vi "NI-DAQmx.vi"() -> (15 "error out":errorcluster)   [LabVIEW 2013]
uses:
  <vilib>/DAQmx/read.llb/DAQmx Read (Analog 2D DBL NChan NSamp).vi
  Globals/Meas_global.vi
  PWA/PWAtasksGLOBAL.vi
  <vilib>/DAQmx/configure/timing.llb/DAQmx Timing (Sample Clock).vi
  <vilib>/DAQmx/miscellaneous.llb/DAQmx Fill In Error Info.vi
  <resource>/objmgr/daqmx.rc
panel:
  out "CurrReadPos 2":dbl=1024.0
  out "AvailSampPerChan 2":u32
  out "TotalSampPerChanAcquired 2":dbl=1024.0
  out "AuditTrail":string[](array[string])
  out "TotalSampPerChanAcquired":dbl=1024.0
  out "AvailSampPerChan":u32
  out "CurrReadPos":dbl=1024.0
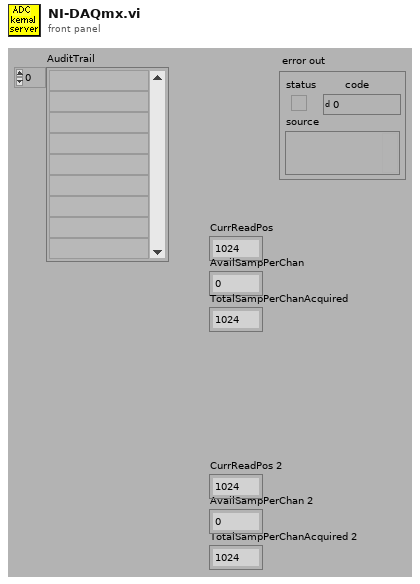
[diagram p1: front panel]
types:
  T1 = typedef "Ch_and_Spans.ctl" = cluster{"high limit (10V)":sgl, "low limit (-10V)":sgl, "Ch No":i16, "Var name":string, "Use Latest Calib":bool, "DAQmx Chan":tag}
  T2 = typedef "LDA_Setup.ctl" = cluster{"dimensions":enum16{"1D", "2D"}, "Analogue Freq Multiplier":dbl}
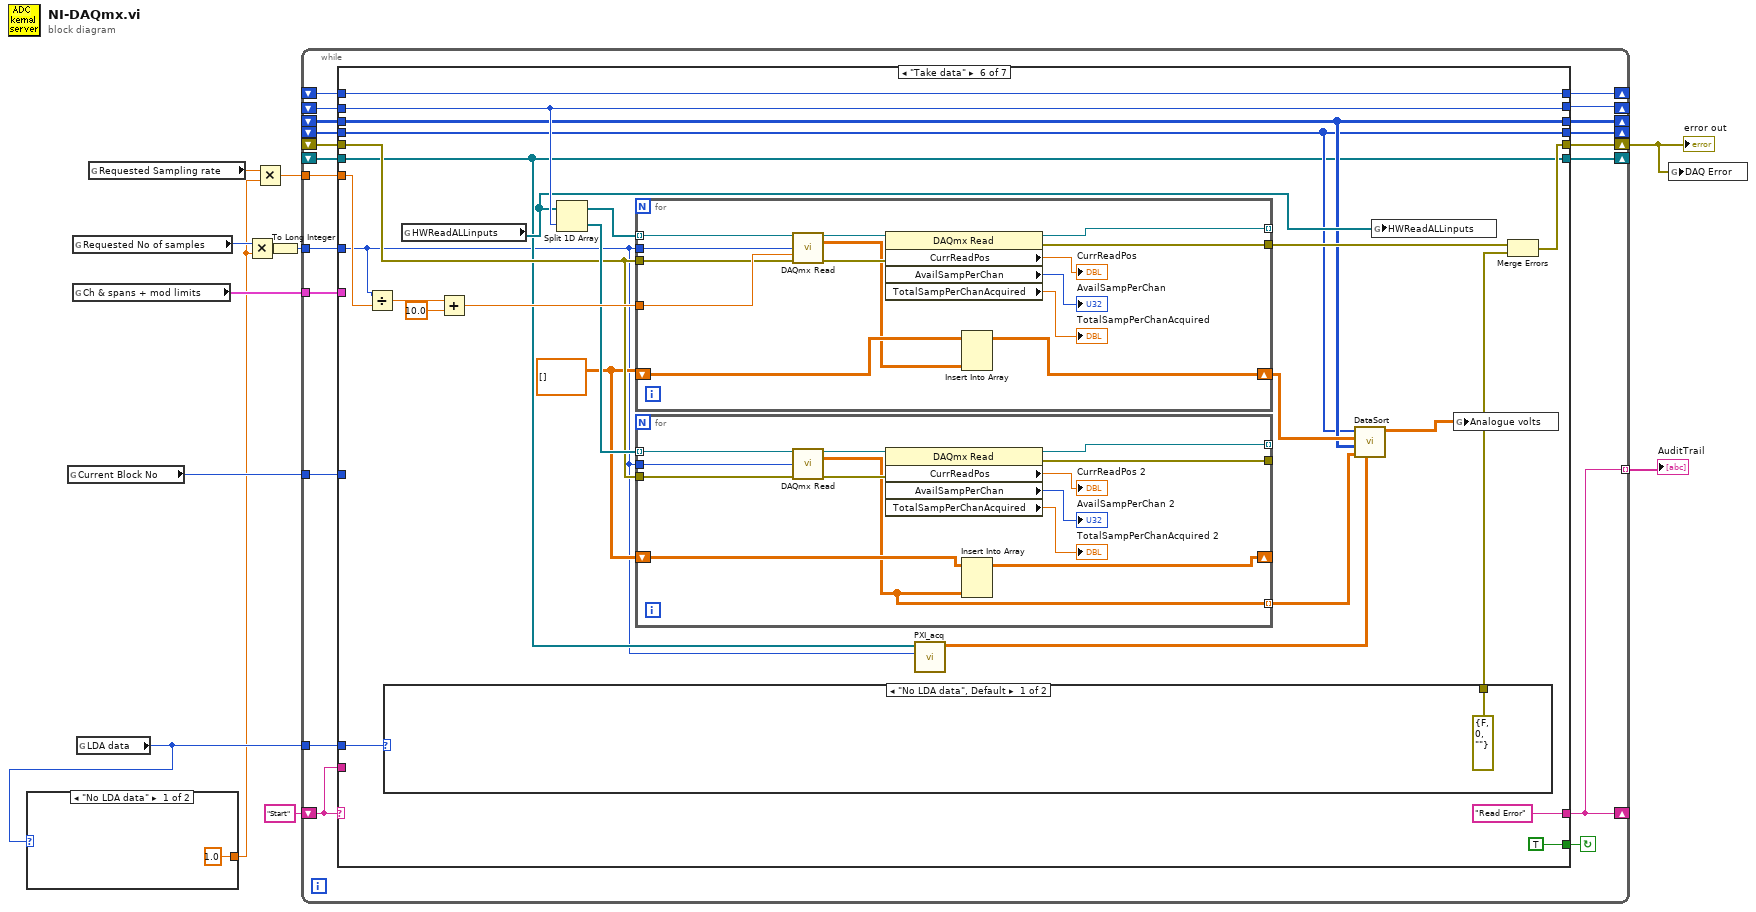
[diagram p0: block diagram]
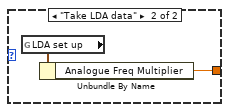
[diagram p2: hidden frame]
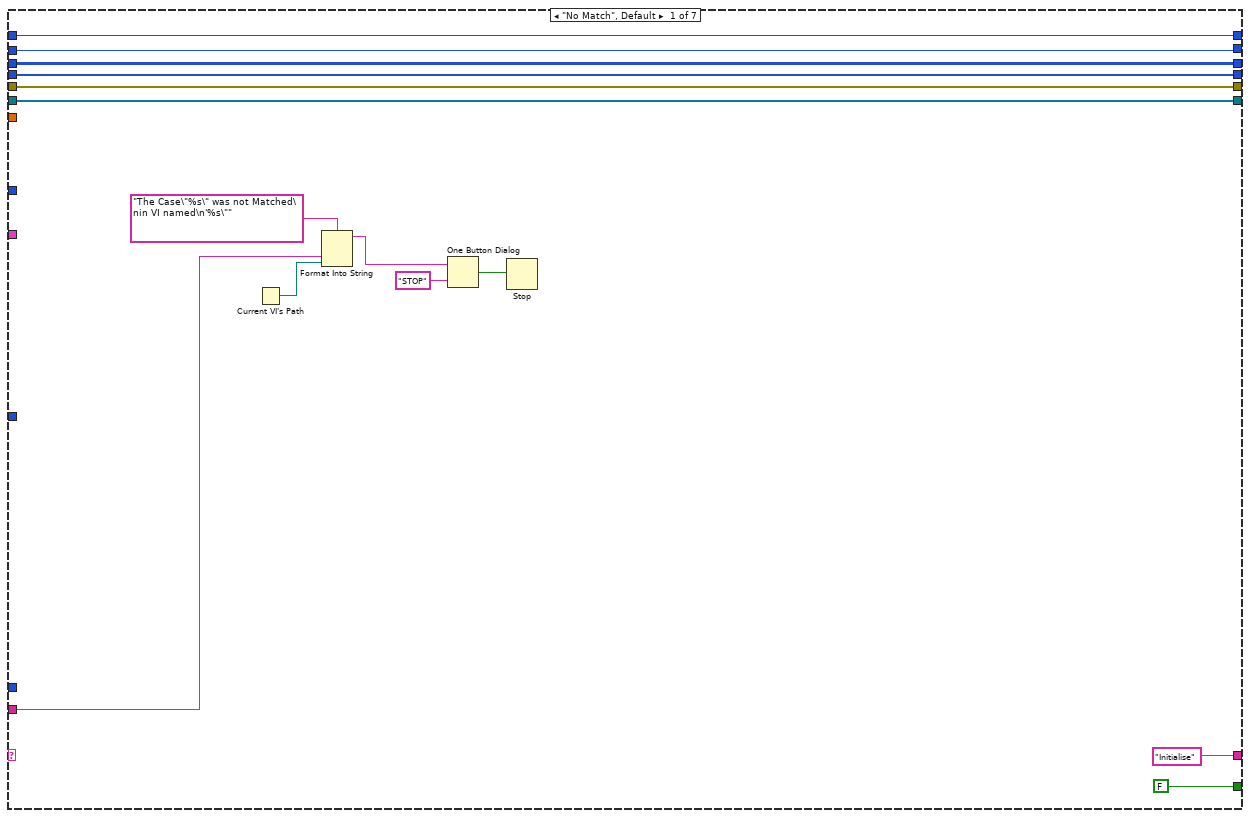
[diagram p3: hidden frame]
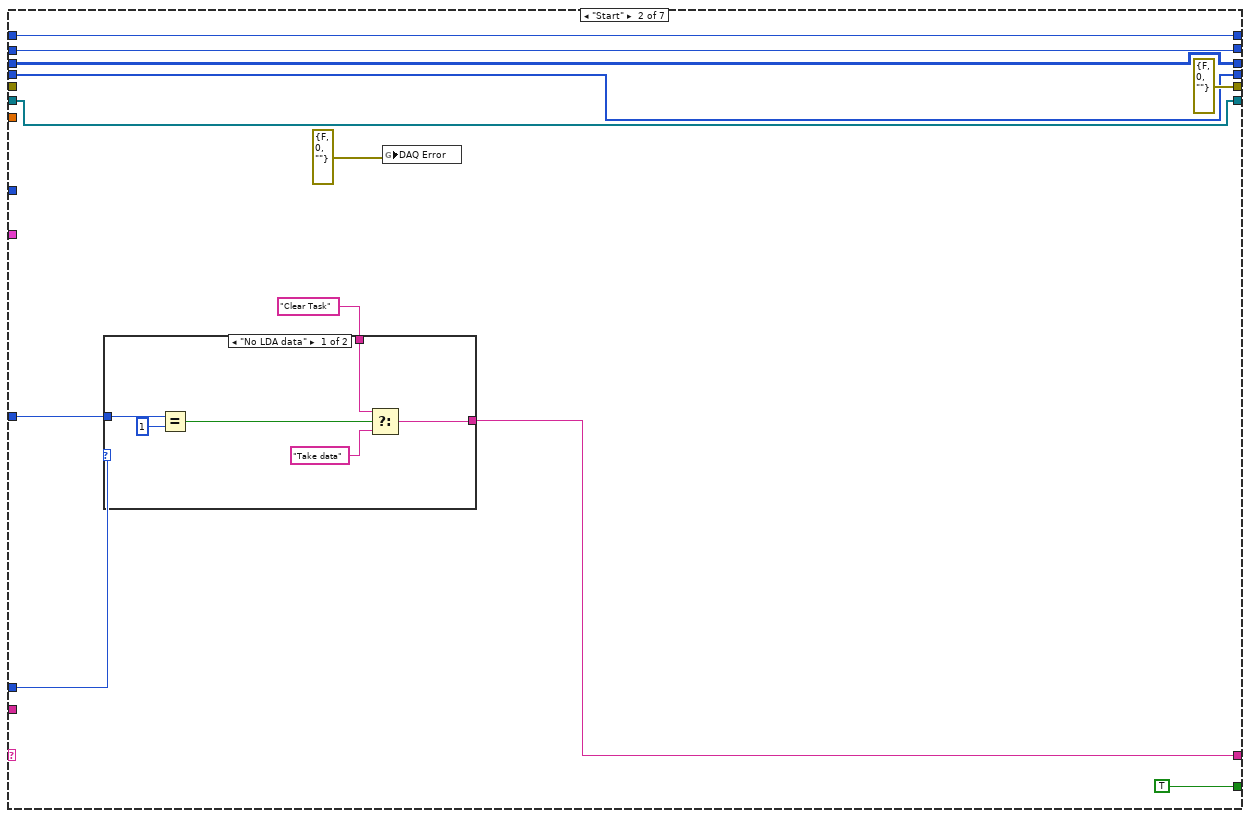
[diagram p4: hidden frame]
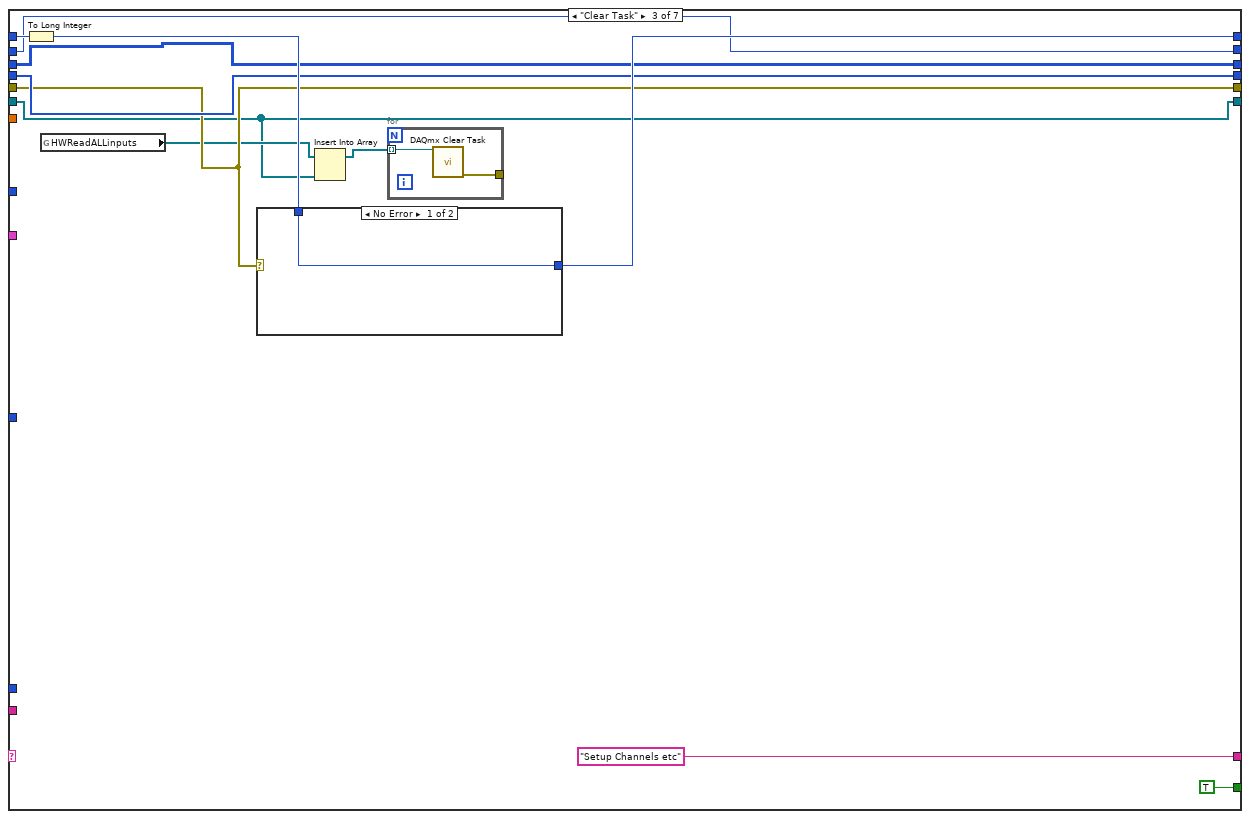
[diagram p6: hidden frame]
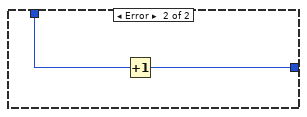
[diagram p7: hidden frame]
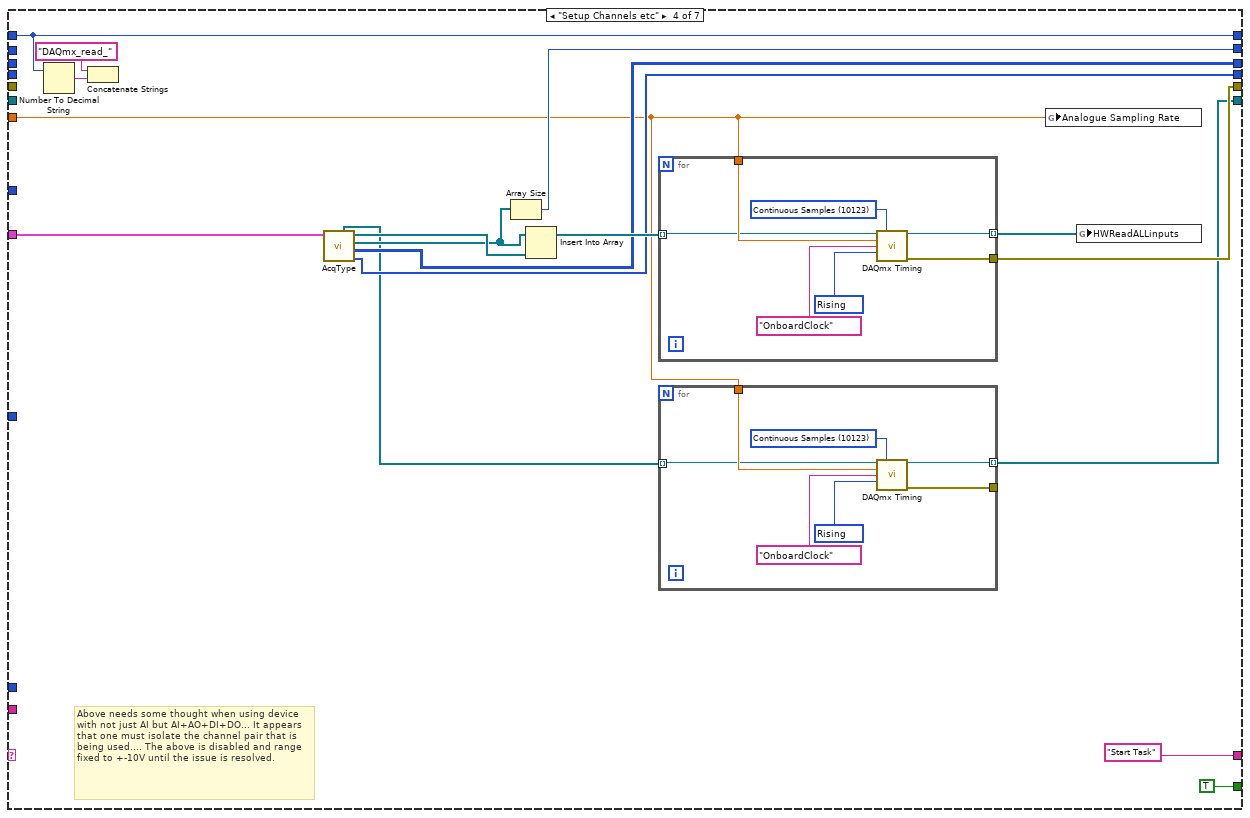
[diagram p8: hidden frame]
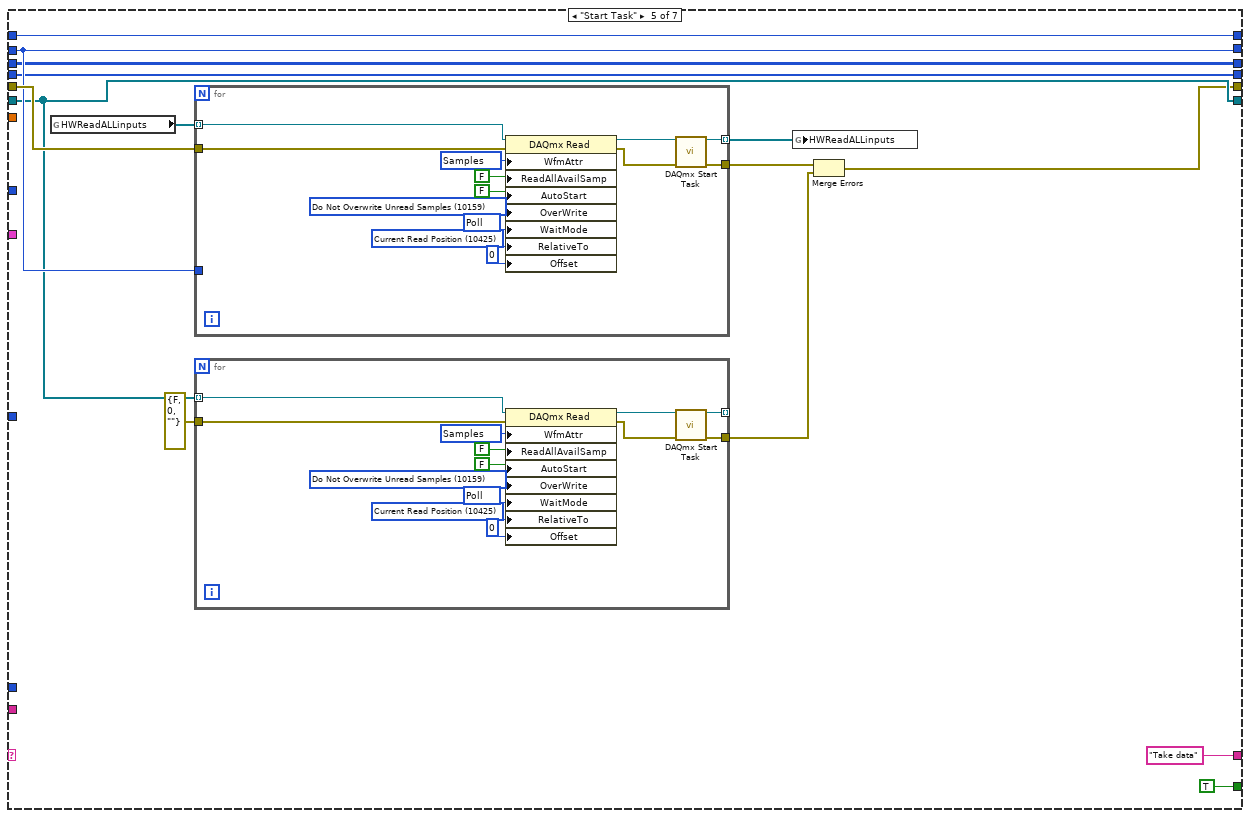
[diagram p9: hidden frame]
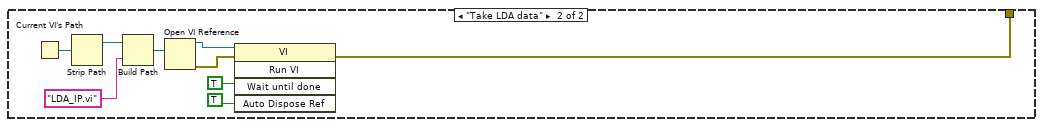
[diagram p10: hidden frame]
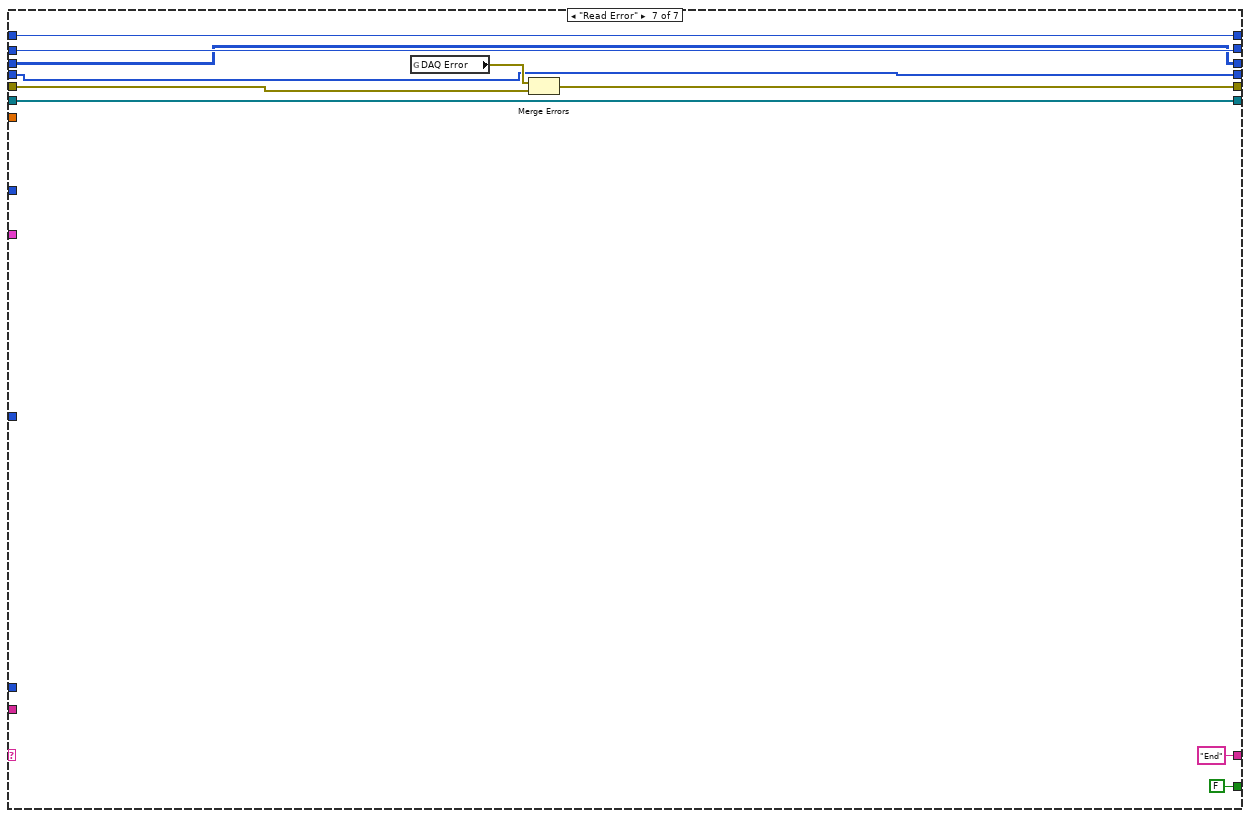
[diagram p11: hidden frame]
diagram:
  n1 = global read "Meas_global.vi" "Current Block No"() -> (w10:i32)
  n2 = global read "Meas_global.vi" "Requested No of samples"() -> (w6:i32)
  n3 = global read "Meas_global.vi" "Ch & spans + mod limits"() -> (w11:T1[])
  n4 = global read "Meas_global.vi" "LDA data"() -> (w8:enum16{"No LDA data", "Take LDA data"})
  n5 = case shown="\"No LDA data\"" w8 {
    tunnel: [1.0 ("Analogue Freq Multiplier") w14] -> w4
    frame "No LDA data" {
    }
    frame "Take LDA data" {
      n6 = global read "Meas_global.vi" "LDA set up"() -> (w15:T2)
      n7 = Unbundle By Name(w15) -> ("Analogue Freq Multiplier"=w14:dbl)
    }
  }
  n8 = global read "Meas_global.vi" "Requested Sampling rate"() -> (w5:dbl)
  n9 = Multiply(x=w6, y=w4) -> (x*y=w7:dbl)
  n10 = Multiply(x=w5, y=w4) -> (x*y=w3:dbl)
  n11 = To Long Integer(number=w7) -> (32bit integer=w2:i32)
  n12 = while {
    shift-left: "Start" -> [w34]
    shift-right: [w24] -> _
    shift-right: [w28] -> w9
    shift-left: _ -> [w33]
    tunnel: w3 -> [w32]
    tunnel: w2 -> [w31]
    tunnel: w10 -> [w30]
    tunnel: w11 -> [w29]
    shift-right: [w27] -> _
    shift-left: _ -> [w26]
    tunnel: w8 -> [w25]
    tunnel: [w24] -> w1 mode=indexing
    shift-right: [w23] -> _
    shift-left: _ -> [w22]
    shift-right: [w21] -> _
    shift-left: _ -> [w20]
    shift-right: [w19] -> _
    shift-left: _ -> [w18]
    shift-right: [w17] -> _
    shift-left: _ -> [w16]
    stop <- w35 continue-if-true
    n13 = case shown="\"Take data\"" w34 {
      tunnel: [FALSE TRUE TRUE TRUE TRUE TRUE FALSE] -> w35
      tunnel: ["Initialise" w59 "Setup Channels etc" "Start Task" "Take data" "Read Error" "End" ("f")] -> w24
      tunnel: w34 -> [w44 _ _ _ _ _ _]
      tunnel: [w41 errorcluster {"status"=FALSE, "code"=0, "source"=""} ("error out") w72 w101 w117 w171 w226] -> w28
      tunnel: w33 -> [w41 _ w72 _ w128 w167 w227]
      tunnel: w32 -> [_ _ _ w87 _ w178 _]
      tunnel: w31 -> [_ _ _ _ _ w158 _]
      tunnel: w30 -> [_ w56 _ _ _ _ _]
      tunnel: w29 -> [_ _ _ w96 _ _ _]
      tunnel: [w40 w58 w78 w95 w126 w179 w225] -> w27
      tunnel: w26 -> [w40 w58 w77 w95 w126 w179 w225]
      tunnel: w25 -> [_ w55 _ _ _ w174 _]
      tunnel: [w39 w53 w75 w90 w124 w170 w222] -> w23
      tunnel: w22 -> [w39 w53 w75 _ w124 w170 w222]
      tunnel: [w38 w52 w74 w92 w123 w163 w221] -> w21
      tunnel: w20 -> [w38 w52 w74 _ w123 w163 w221]
      tunnel: [w37 w51 w73 w89 w122 w162 w220] -> w19
      tunnel: w18 -> [w37 w51 w73 _ w122 w162 w220]
      tunnel: [w36 w50 w69 w86 w121 w159 w219] -> w17
      tunnel: w16 -> [w36 w50 w69 _ w121 w159 w219]
      frame "No Match", Default {
        n14 = Current VI's Path() -> (path=w43:path)
        n15 = Format Into String(format string="The Case\"%s\" was not Matched\nin VI named\n'%s\"" ("Format String"), w44, w43) -> (resulting string=w47:string)  [unwired: 2 in, 1 out]
        n16 = One Button Dialog(message=w47, button name ("OK")="STOP") -> (true=w45:bool)
        n17 = Stop(stop? (T)=w45) -> ()
      }
      frame "Start" {
        n18 = case shown="\"No LDA data\"" w55 {
          tunnel: "Clear Task" -> [w67 w68]
          tunnel: [w65 w68] -> w59
          tunnel: w56 -> [w64 _]
          frame "No LDA data" {
            n19 = Equal?(x=w64, y=1) -> (x = y?=w62:bool)
            n20 = Select(t=w67, s=w62, f="Take data") -> (s? t:f=w65:string)
          }
          frame "Take LDA data" {
          }
        }
        n21 = global write "Meas_global.vi" "DAQ Error"(errorcluster {"status"=FALSE, "code"=0, "source"=""} ("DAQ Error")) -> ()
      }
      frame "Clear Task" {
        n22 = To Long Integer(number=w77) -> (32bit integer=w76:i32)
        n23 = global read "PWAtasksGLOBAL.vi" "HWReadALLinputs"() -> (w71:refnum<k21>[])
        n24 = case shown="No Error" w72 {
          tunnel: [w83 w84] -> w78
          tunnel: w76 -> [w83 w85]
          frame No Error {
          }
          frame Error {
            n25 = Increment(x=w85) -> (x+1=w84:i32)
          }
        }
        n26 = Insert Into Array(array=w71, new element=w69) -> (w70:refnum<k21>[])  [unwired: 1 in]
        n27 = for {
          tunnel: w70 -> [w82] mode=indexing
          tunnel: [w81] -> _
          n28 = call <vilib>:"DAQmx Clear Task.vi"("task in"=w82) -> ("error out"=w81:errorcluster)  [unwired: 1 in, 13 out]
        }
      }
      frame "Setup Channels etc" {
        # "Above needs some thought when using device with not just AI but AI+AO+DI+DO... It appears that one must isolate the channel pair that is being used.... The above is disabled and range fixed to +-10V until the issue is resolved."
        n29 = Number To Decimal String(number=w95) -> (decimal integer string=w97:string)  [unwired: 1 in]
        n30 = Concatenate Strings("DAQmx_read_" ("new task name"), w97) -> ()  [unwired: 1 out]
        n31 = call "AcqType.vi"("Ch & spans + mod limits"=w96) -> ("cDAQ i"=w89:i32[], "eDAQ i"=w92:i32[][], "cDAQ tasks"=w91:refnum<k21>[], "eDAQ tasks"=w93:refnum<k21>[], "PXIs"=w88:refnum<k21>[])  [unwired: 5 in, 1 out]
        n32 = Array Size(array=w91) -> (size(s)=w90:i32)
        n33 = Insert Into Array(array=w91, new element=w93) -> (w94:refnum<k21>[])  [unwired: 1 in]
        n34 = for {
          tunnel: [w115] -> w101
          tunnel: [w114] -> w100 mode=indexing
          tunnel: w87 -> [w111]
          tunnel: w94 -> [w110] mode=indexing
          w113 = 10280 items=["Rising"=10280, "Falling"=10171] ("active edge")
          w116 = 10123 items=["Finite Samples"=10178, "Continuous Samples"=10123, "Hardware Timed Single Point"=12522] ("sample mode")
          n35 = call-poly <vilib>:"DAQmx Timing.vi"("task/channels in"=w110, "sample mode"=w116, "rate"=w111, "source"=tag "OnboardClock", "active edge"=w113) -> ("task out"=w114:refnum<k21>, "error out"=w115:errorcluster)  [unwired: 2 in, 7 out]
        }
        n36 = for {
          tunnel: [w108] -> _
          tunnel: [w107] -> w86 mode=indexing
          tunnel: w87 -> [w104]
          tunnel: w88 -> [w103] mode=indexing
          w106 = 10280 items=["Rising"=10280, "Falling"=10171] ("active edge")
          w109 = 10123 items=["Finite Samples"=10178, "Continuous Samples"=10123, "Hardware Timed Single Point"=12522] ("sample mode")
          n37 = call-poly <vilib>:"DAQmx Timing.vi"("task/channels in"=w103, "sample mode"=w109, "rate"=w104, "source"=tag "OnboardClock", "active edge"=w106) -> ("task out"=w107:refnum<k21>, "error out"=w108:errorcluster)  [unwired: 2 in, 7 out]
        }
        n38 = global write "Meas_global.vi" "Analogue Sampling Rate"(w87) -> ()
        n39 = global write "PWAtasksGLOBAL.vi" "HWReadALLinputs"(w100) -> ()
      }
      frame "Start Task" {
        n40 = global read "PWAtasksGLOBAL.vi" "HWReadALLinputs"() -> (w129:refnum<k21>[])
        n41 = for {
          tunnel: w129 -> [w156] mode=indexing
          tunnel: w128 -> [w155]
          tunnel: [w152] -> w119
          tunnel: [w151] -> w125 mode=indexing
          tunnel: w124 -> [_]
          w145 = 10425 items=["First Sample"=10424, "Current Read Position"=10425, "Reference Trigger"=10426, "First Pretrigger Sample"=10427, "Most Recent Sample"=10428] ("RelativeTo")
          w146 = 12524 items=["Wait For Interrupt"=12523, "Poll"=12524, "Yield"=12525, "Sleep"=12547] ("WaitMode")
          w147 = 10159 items=["Overwrite Unread Samples"=10252, "Do Not Overwrite Unread Samples"=10159] ("OverWrite")
          w149 = 10287 items=["Samples"=10287, "Samples and Timing"=10140, "Samples, Timing, and Attributes"=10141] ("WfmAttr")
          n42 = property class="DAQmx Read"(reference=w156, error in=w155, "WfmAttr"=w149, "ReadAllAvailSamp"=FALSE, "AutoStart"=FALSE, "OverWrite"=w147, "WaitMode"=w146, "RelativeTo"=w145, "Offset"=0) -> (reference out=w153:refnum<k21>, error out=w154:errorcluster)
          n43 = call <vilib>:"DAQmx Start Task.vi"("task/channels in"=w153, "error in"=w154) -> ("task out"=w151:refnum<k21>, "error out"=w152:errorcluster)  [unwired: 12 out]
        }
        n44 = for {
          tunnel: w121 -> [w143] mode=indexing
          tunnel: errorcluster {"status"=FALSE, "code"=0, "source"=""} ("error IO") -> [w142]
          tunnel: [w139] -> w118
          tunnel: [w138] -> _ mode=indexing
          w132 = 10425 items=["First Sample"=10424, "Current Read Position"=10425, "Reference Trigger"=10426, "First Pretrigger Sample"=10427, "Most Recent Sample"=10428] ("RelativeTo")
          w133 = 12524 items=["Wait For Interrupt"=12523, "Poll"=12524, "Yield"=12525, "Sleep"=12547] ("WaitMode")
          w134 = 10159 items=["Overwrite Unread Samples"=10252, "Do Not Overwrite Unread Samples"=10159] ("OverWrite")
          w136 = 10287 items=["Samples"=10287, "Samples and Timing"=10140, "Samples, Timing, and Attributes"=10141] ("WfmAttr")
          n45 = property class="DAQmx Read"(reference=w143, error in=w142, "WfmAttr"=w136, "ReadAllAvailSamp"=FALSE, "AutoStart"=FALSE, "OverWrite"=w134, "WaitMode"=w133, "RelativeTo"=w132, "Offset"=0) -> (reference out=w140:refnum<k21>, error out=w141:errorcluster)
          n46 = call <vilib>:"DAQmx Start Task.vi"("task/channels in"=w140, "error in"=w141) -> ("task out"=w138:refnum<k21>, "error out"=w139:errorcluster)  [unwired: 12 out]
        }
        n47 = global write "PWAtasksGLOBAL.vi" "HWReadALLinputs"(w125) -> ()
        n48 = Merge Errors(w119, w118) -> (w117:errorcluster)
      }
      frame "Take data" {
        w161 = dbl[][] [] ("data")
        n49 = Divide(x=w158, y=w178) -> (x/y=w177:dbl)
        n50 = case shown="\"No LDA data\", Default" w174 {
          tunnel: [errorcluster {"status"=FALSE, "code"=0, "source"=""} ("error out") w210] -> w173
          frame "No LDA data", Default {
          }
          frame "Take LDA data" {
            n51 = Current VI's Path() -> (path=w212:path)
            n52 = Strip Path(path=w212) -> (stripped path=w211:path)  [unwired: 1 out]
            n53 = Build Path(base path=w211, name or relative path="LDA_IP.vi") -> (appended path=w213:path)
            n54 = Open VI Reference(vi path=w213) -> (vi reference=w216:refnum<vi>, error out=w217:errorcluster)  [unwired: 5 in]
            n55 = invoke class="VI" method="Run VI"(reference=w216, error in=w217, "Wait until done"=TRUE ("Wait Until Done"), "Auto Dispose Ref"=TRUE ("Wait until done")) -> (error out=w210:errorcluster)  [unwired: 1 in, 4 out]
          }
        }
        n56 = global read "PWAtasksGLOBAL.vi" "HWReadALLinputs"() -> (w166:refnum<k21>[])
        n57 = Add(x=w177, y=10.0) -> (x+y=w175:dbl)
        n58 = Split 1D Array(array=w166, index=w170) -> (first subarray=w169:refnum<k21>[], second subarray=w168:refnum<k21>[])
        n59 = for {
          tunnel: w167 -> [w195]
          tunnel: [w205] -> _ mode=indexing
          tunnel: w169 -> [w196] mode=indexing
          tunnel: w175 -> [w202]
          tunnel: [w201] -> w172
          tunnel: w158 -> [w200]
          shift-right: [w197] -> w165
          shift-left: w161 -> [w199]
          n60 = call-poly <vilib>:"DAQmx Read.vi"("task/channels in"=w196, "number of samples per channel"=w200, "timeout"=w202, "error in"=w195) -> ("task out"=w206:refnum<k21>, "data"=w198:dbl[][], "error out"=w203:errorcluster)  [unwired: 9 out]
          n61 = property class="DAQmx Read"(reference=w206, error in=w203) -> (reference out=w205:refnum<k21>, error out=w201:errorcluster, "CurrReadPos"=→"CurrReadPos":dbl, "AvailSampPerChan"=→"AvailSampPerChan":u32, "TotalSampPerChanAcquired"=→"TotalSampPerChanAcquired":dbl)
          n62 = Insert Into Array(array=w199, new element=w198) -> (w197:dbl[][])  [unwired: 2 in]
        }
        n63 = for {
          tunnel: w167 -> [w185]
          tunnel: [w191] -> _ mode=indexing
          tunnel: w168 -> [w186] mode=indexing
          tunnel: [w188] -> _
          tunnel: w158 -> [w187]
          shift-right: [w183] -> _
          shift-left: w161 -> [w184]
          tunnel: [w182] -> w160 mode=indexing
          n64 = call-poly <vilib>:"DAQmx Read.vi"("task/channels in"=w186, "number of samples per channel"=w187, "error in"=w185) -> ("task out"=w192:refnum<k21>, "data"=w182:dbl[][], "error out"=w189:errorcluster)  [unwired: 1 in, 9 out]
          n65 = property class="DAQmx Read"(reference=w192, error in=w189) -> (reference out=w191:refnum<k21>, error out=w188:errorcluster, "CurrReadPos"=→"CurrReadPos 2":dbl, "AvailSampPerChan"=→"AvailSampPerChan 2":u32, "TotalSampPerChanAcquired"=→"TotalSampPerChanAcquired 2":dbl)
          n66 = Insert Into Array(array=w184, new element=w182) -> (w183:dbl[][])  [unwired: 2 in]
        }
        n67 = call "PXI_acq.vi"("Sampels/Ch"=w158, "Tasks"=w159) -> ("Data"=w157:dbl[][][])  [unwired: 9 in]
        n68 = call "DataSort.vi"("PXI"=w157, "eDAQ"=w160, "eDAQ i"=w163, "cDAQ"=w165, "cDAQ i"=w162) -> ("Data Out"=w164:dbl[][])  [unwired: 6 in]
        n69 = global write "PWAtasksGLOBAL.vi" "HWReadALLinputs"(w166) -> ()
        n70 = global write "Meas_global.vi" "Analogue volts"(w164) -> ()
        n71 = Merge Errors(w172, w173) -> (w171:errorcluster)
      }
      frame "Read Error" {
        n72 = global read "Meas_global.vi" "DAQ Error"() -> (w228:errorcluster)
        n73 = Merge Errors(w228, w227) -> (w226:errorcluster)
      }
    }
  }
  "error out" <- w9
  "AuditTrail" <- w1
  n74 = global write "Meas_global.vi" "DAQ Error"(w9) -> ()
